vi "setZkAndDofInGroups.vi"(8 "error in (no error)":errorcluster, 9 "DOF in Groups":T1={"M2 Hexapod"=[FALSE, FALSE, FALSE, FALSE, FALSE], "Cam Hexapod "=[FALSE, FALSE, FALSE, FALSE, FALSE], "M1M3 Bending Mode"=[FALSE, FALSE, FALSE, FALSE, FALSE, FALSE, FALSE, FALSE, FALSE, FALSE, FALSE, FALSE, FALSE, FALSE, FALSE, FALSE, FALSE, FALSE, FALSE, FALSE], "M2 Bending Mode"=[FALSE, FALSE, FALSE, FALSE, FALSE, FALSE, FALSE, FALSE, FALSE, FALSE, FALSE, FALSE, FALSE, FALSE, FALSE, FALSE, FALSE, FALSE, FALSE, FALSE]}, 10 "zn3Idx":bool[](array[boolean])=[FALSE, FALSE, FALSE, FALSE, FALSE, FALSE, FALSE, FALSE, FALSE, FALSE, FALSE, FALSE, FALSE, FALSE, FALSE, FALSE, FALSE, FALSE, FALSE], 11 "OptStateEsti in":refnum<class "OptStateEsti.lvclass">) -> (0 "error out":errorcluster, 3 "OptStateEsti out":refnum<class "OptStateEsti.lvclass">)   [LabVIEW 2016, in "OptStateEsti.lvclass"]
doc: "Set the index array of Zk and DOF in groups (M2 hexapod, camera hexapod, M1M3 bending mode, M2 bending mode)."
uses:
  OptStateEsti.lvclass
  OptStateEsti.lvclass/OptStateEsti.ctl
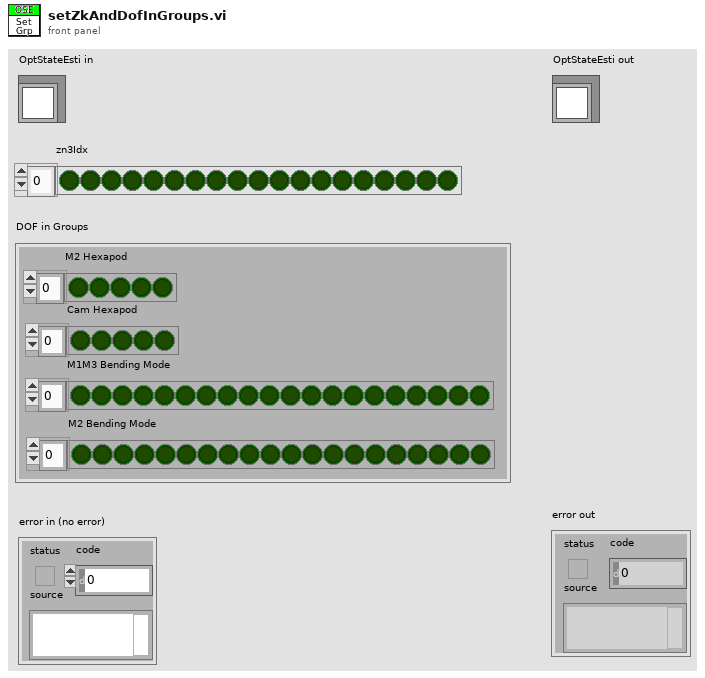
[diagram p1: front panel]
types:
  T1 = cluster{"M2 Hexapod":bool[], "Cam Hexapod ":bool[], "M1M3 Bending Mode":bool[], "M2 Bending Mode":bool[]}
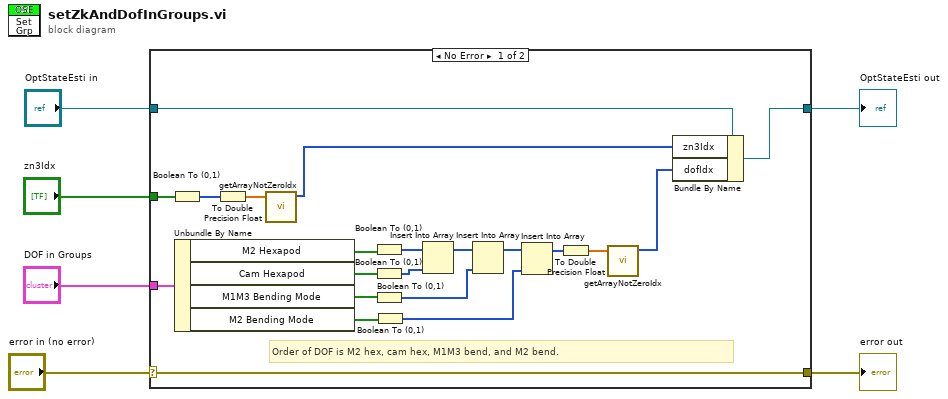
[diagram p0: block diagram]
diagram:
  n1 = case shown="No Error" "error in (no error)" {
    selector: "error in (no error)" -> [w27 w29]
    tunnel: [w27 w29] -> w5
    tunnel: [w21 w28] -> w3
    tunnel: "OptStateEsti in" -> [w22 w28]
    tunnel: "zn3Idx" -> [w26 _]
    tunnel: "DOF in Groups" -> [w20 _]
    frame No Error {
      # "Order of DOF is M2 hex, cam hex, M1M3 bend, and M2 bend."
      n2 = Boolean To (0,1)(Boolean=w26) -> (0, 1=w25:i16[])
      n3 = Unbundle By Name(w20) -> ("M2 Hexapod"=w7:bool[], "Cam Hexapod"=w19:bool[], "M1M3 Bending Mode"=w18:bool[], "M2 Bending Mode"=w17:bool[])
      n4 = To Double Precision Float(number=w25) -> (double precision float=w24:dbl[])
      n5 = call "getArrayNotZeroIdx.vi"("Array"=w24) -> ("Index Array"=w23:i32[])  [unwired: 10 in]
      n6 = Boolean To (0,1)(Boolean=w7) -> (0, 1=w16:i16[])
      n7 = Boolean To (0,1)(Boolean=w19) -> (0, 1=w15:i16[])
      n8 = Boolean To (0,1)(Boolean=w18) -> (0, 1=w13:i16[])
      n9 = Boolean To (0,1)(Boolean=w17) -> (0, 1=w11:i16[])
      n10 = Insert Into Array(array=w16, new element=w15) -> (w14:i16[])  [unwired: 1 in]
      n11 = Insert Into Array(array=w14, new element=w13) -> (w12:i16[])  [unwired: 1 in]
      n12 = Insert Into Array(array=w12, new element=w11) -> (w10:i16[])  [unwired: 1 in]
      n13 = To Double Precision Float(number=w10) -> (double precision float=w9:dbl[])
      n14 = call "getArrayNotZeroIdx.vi"("Array"=w9) -> ("Index Array"=w8:i32[])  [unwired: 10 in]
      n15 = Bundle By Name(cluster=w22, "zn3Idx"=w23, "dofIdx"=w8) -> (w21:refnum<class "OptStateEsti.lvclass">)
    }
    frame Error {
    }
  }
  "error out" <- w5
  "OptStateEsti out" <- w3
